vi "NB_ReadWriteAttribute_IPE.vi"(8 "error in (no error)":errorcluster, 11 "object in":refnum<class "NativeBaseTemplate_4x4x4.lvclass">) -> (0 "error out":errorcluster, 3 "object out":refnum<class "NativeBaseTemplate_4x4x4.lvclass">)   [LabVIEW 2020, in "NativeBaseTemplate_4x4x4.lvclass"]
uses:
  <resource>/Framework/Providers/Open_GDS/ClassProviders/Provider_LvNativeClass/Templates/NativeBaseTemplate_4x4x4/NativeBaseTemplate_4x4x4.lvclass
  <resource>/Framework/Providers/Open_GDS/ClassProviders/Provider_LvNativeClass/Templates/NativeBaseTemplate_4x4x4/NativeBaseTemplate_4x4x4.lvclass/NativeBaseTemplate_4x4x4.ctl
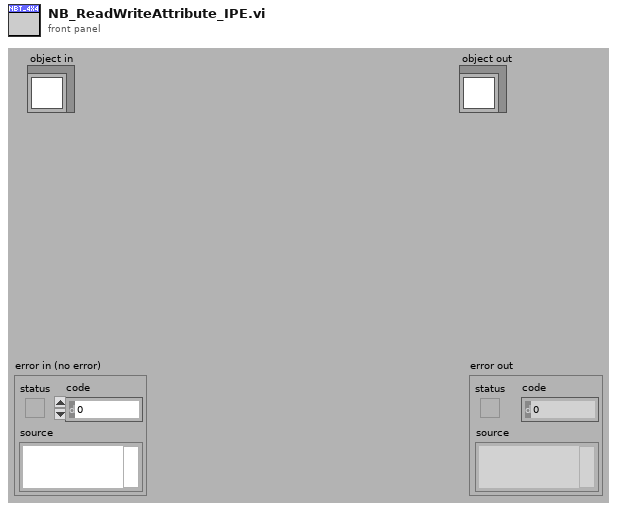
[diagram p1: front panel]
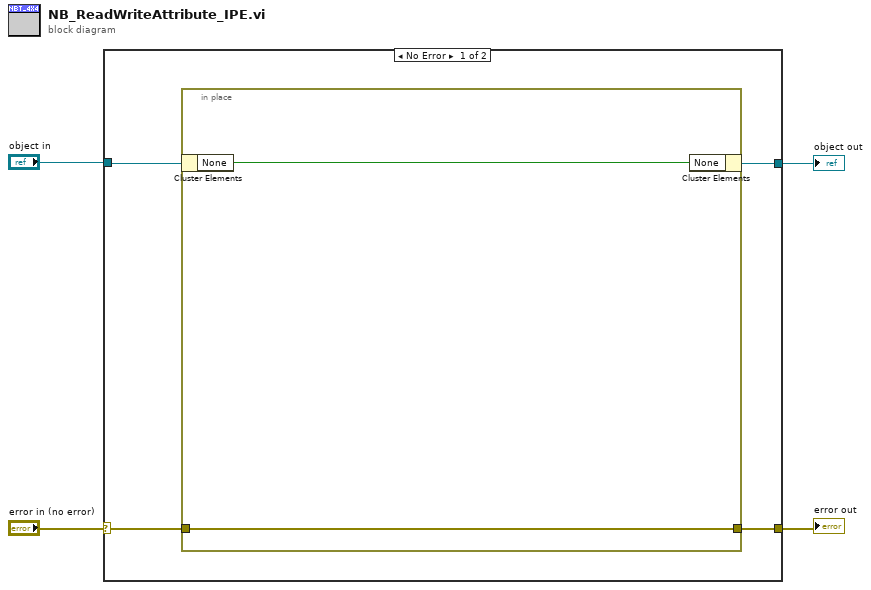
[diagram p0: block diagram]
diagram:
  n1 = case shown="No Error" "error in (no error)" {
    selector: "error in (no error)" -> [w5 w12]
    tunnel: [w6 w12] -> w2
    tunnel: [w7 w11] -> w1
    tunnel: "object in" -> [w8 w11]
    frame No Error {
      n2 = in-place {
        in-place-border: [w9] -> w6
        in-place-border: w5 -> [w9]
        n3 = in-place-cluster #1(w8) -> ("None"=w10:bool)
        n4 = in-place-cluster #1("None"=w10) -> (w7:refnum<class "NativeBaseTemplate_4x4x4.lvclass">)
      }
    }
    frame Error {
    }
  }
  "error out" <- w2
  "object out" <- w1
